vi "Z-Scan.vi"() -> ()   [LabVIEW 2020]
uses:
  <vilib>/LabVIEW Interface for Arduino/Type Defs/Board Type.ctl
  <vilib>/LabVIEW Interface for Arduino/Type Defs/Connection Type.ctl
  <vilib>/Utility/error.llb/DialogType.ctl
  <vilib>/Utility/file.llb/Write Delimited Spreadsheet (string).vi
panel:
  in  "Unidade de medida":bool
  in  "Distancia entre medidas":sgl
  out "Rodando":bool
  in  "Numero de medidas":i32
  in  "Distancia percorrida":sgl
  in  "Measurement Function (0: Period)":i32(ring)=17 items=["Period", "Frequency", "Delay", "Rise Time", "Fall Time", "Positive Duty Cycle", "Negative Duty Cycle", "Positive Pulse Width", "Negative Pulse Width", "Burst Width", "Phase", "Positive Overshoot", "Negative Overshoot", "Vpp", "Amplitude", "Voltage High", "Voltage Low", "Voltage Max", "Voltage Min", "Voltage Mean", "Voltage Mean (cycle)", "Voltage RMS", "Voltage RMS (cycle)", "Area", "Cycle Area", "Positive Edge Count", "Negative Edge Count", "Positive Pulse Count", "Negative Pulse Count", "Total Overshoot"]
  in  "Channel (0: Channel 1)":u16(ring) items=["Channel 1", "Channel 2", "Channel 3", "Channel 4", "Math", "D0", "D1", "D2", "D3", "D4", "D5", "D6", "D7", "D8", "D9", "D10", "D11", "D12", "D13", "D14", "D15", "Reference 1", "Reference 2", "Reference 3", "Reference 4", "Amplitude", "Frequency", "Phase"]
  out "Numero de paradas":sgl
  in  "Sair":bool
  out "Tabela":string[][](table)
  out "?":cluster{dbl[], dbl[]}(graph)
  out "Passos entre medidas":sgl
  out "Numero de passos":sgl
  in  "Z-Scan Automatico":bool
  in  "VISA Tektronix DPO 3052":refnum<visa-resource-name>
  in  "VISA Arduino":refnum<visa-resource-name>
  # "Não interromper a medida em andamento pelo abourt execution(canto superior esquedo), risco de dano ao motor"
  # "Para encontrar a COM: Botão Windows/ Dispositivos e impressoras/ Não especificados"
  # "Para o Software Z-Scan\n1) Selecionar a porta do dispositivo:\n  - VISA Arduino (ver a porta do USB-SERIAL CH340)\n  - Visa Tektronix (USB0::0x0699::.. do DPO 3052)\n2) Seleciona o canal do osciloscópio e o tipo de medida:\n  - Channel (ver no osciloscópio: canal 1 ou 2)\n  - Measurement Function (voltagem max)\n3) Dar RUN (canto esquerdo superior da tela)\n3) Definir os parâmetros de medida:\n  - Unidade de medida\n  - Distância percorrida (2*Z)\n  - Distância entre medidas\n  - Número de medidas (para fazer as médias)\n4) Clicla na tela para validar os dados de entrada\n5) Encontrar o foco pelas teclas direita/esquerda do teclado\n6) Clica \"Iniciar\""
  # "Para a montagem Z-Scan\n1) Conectar o osciloscópio e o arduino ao computador\n2) Ligar a fonte do arduino na tomada\n3) Girar o switch da caixinha"
  # "cm"
  # "mm"
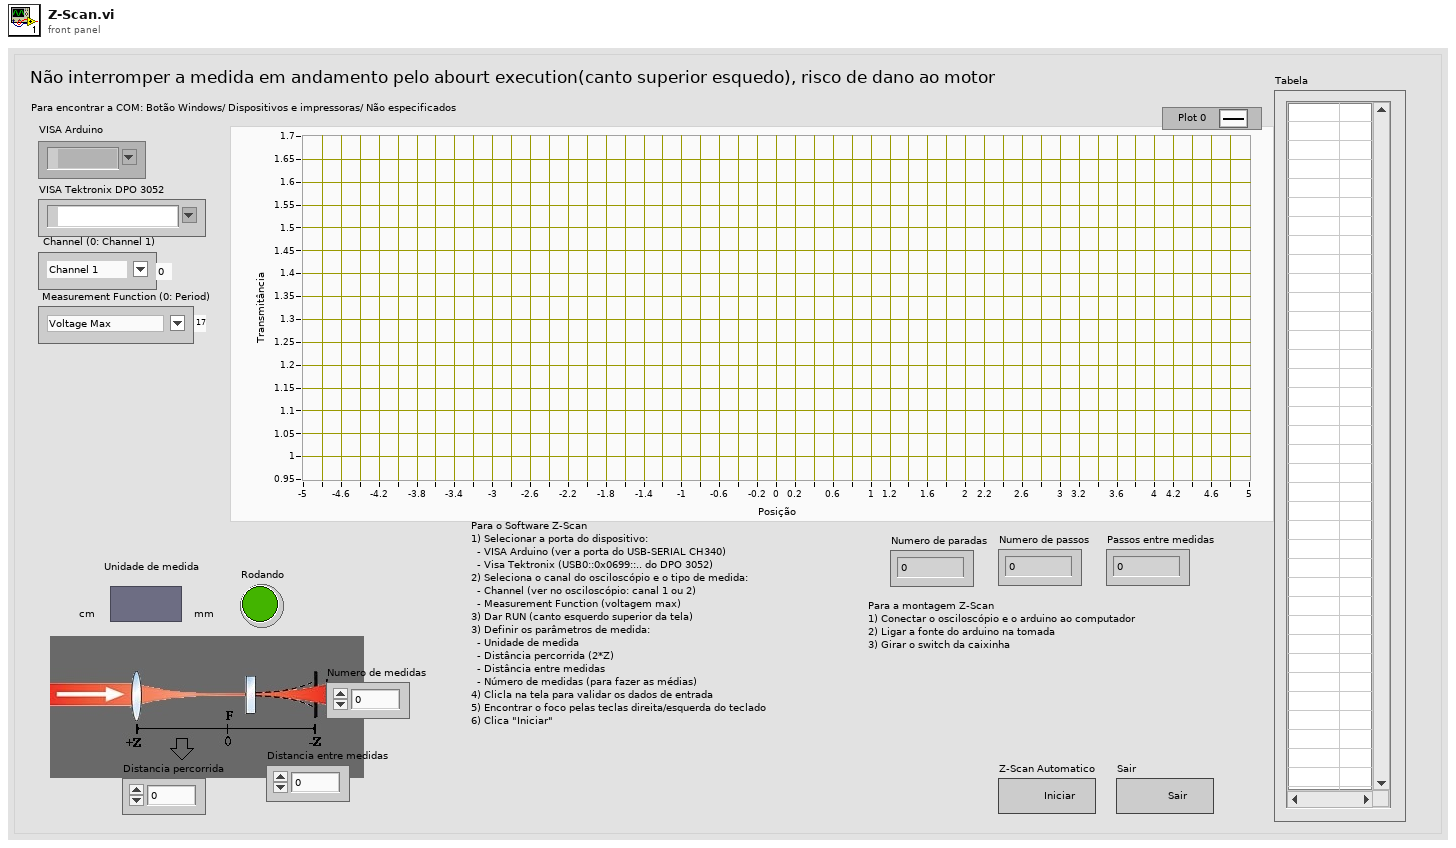
[diagram p1: front panel]
types:
  T1 = typedef "DialogType.ctl" = u16
  T2 = typedef "LabVIEW Interface for Arduino.lvlib/Connection Type.ctl" = enum8{"USB / Serial", "XBEE", "BlueSmirf (Bluetooth)"}
  T3 = typedef "LabVIEW Interface for Arduino.lvlib/Board Type.ctl" = enum16{"Uno", "Dimuelanove w/Atmega 328", "Mega 2560"}
  T4 = typedef "LabVIEW Interface for Arduino.lvlib/Arduino Resource.ctl" = cluster{"VISA resource":refnum<visa-resource-name>, "Board Type":T3, "Connection Type":enum8{"USB / Serial"}, "Bytes Per Packet (15)":u8}
  T5 = typedef "eventvkey.ctl" = enum16{"ASCII", "Enter", "Return", "Shift", "Ctrl", "Alt", "Cmd", "Opt", "Caps", "NumLock", "Clear", "Break", "Up", "Down", "Left", "Right", "Insert", "Delete", "Home", "End", "PageUp", "PageDown", "Escape", "Help", "Pause", "ScrollLock", "F1", "F2", "F3", "F4", "F5", "F6", "F7", "F8", "F9", "F10", "F11", "F12", "F13", "F14", "F15", "F16", "F17", "F18", "F19", "F20", "F21", "F22", "F23", "F24", "Play", "VolumeUp", "VolumeDown", "Mute", "Two Byte Char"}
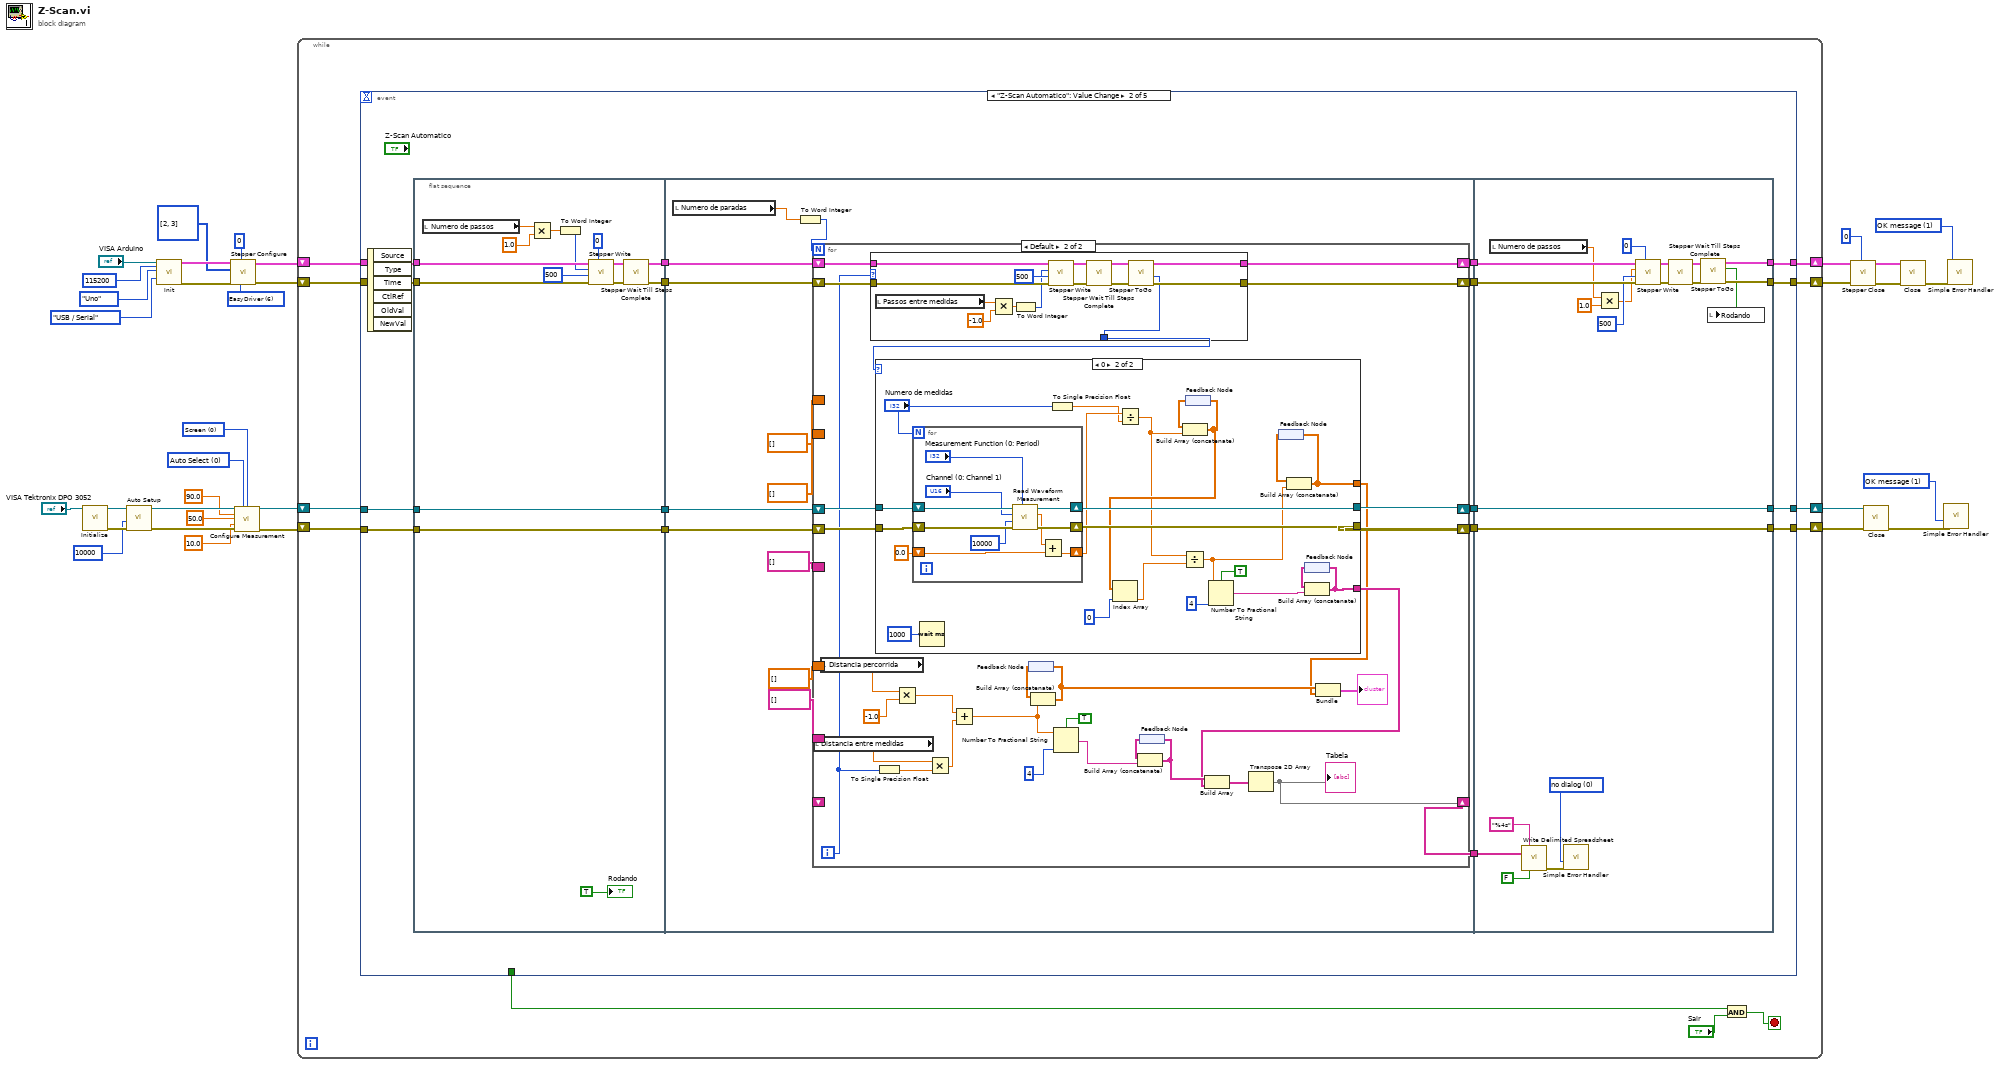
[diagram p0: block diagram]
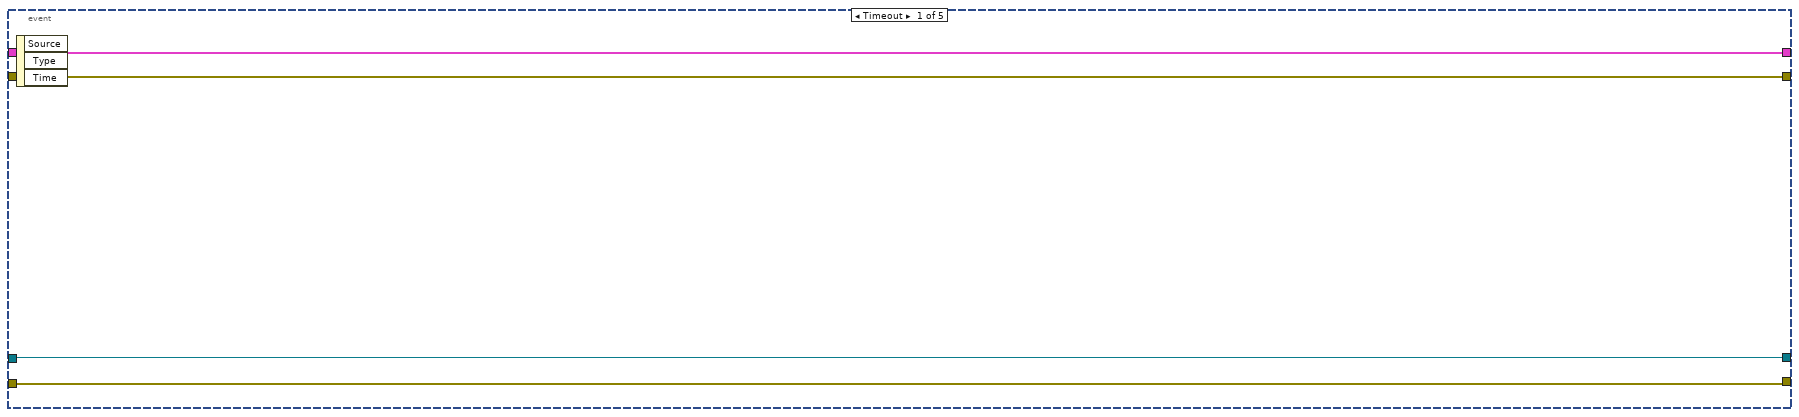
[diagram p2: hidden frame]
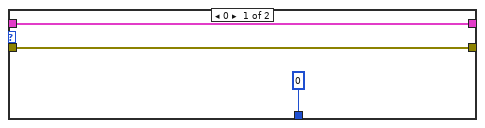
[diagram p3: hidden frame]
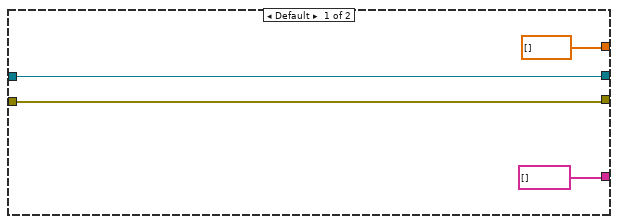
[diagram p4: hidden frame]
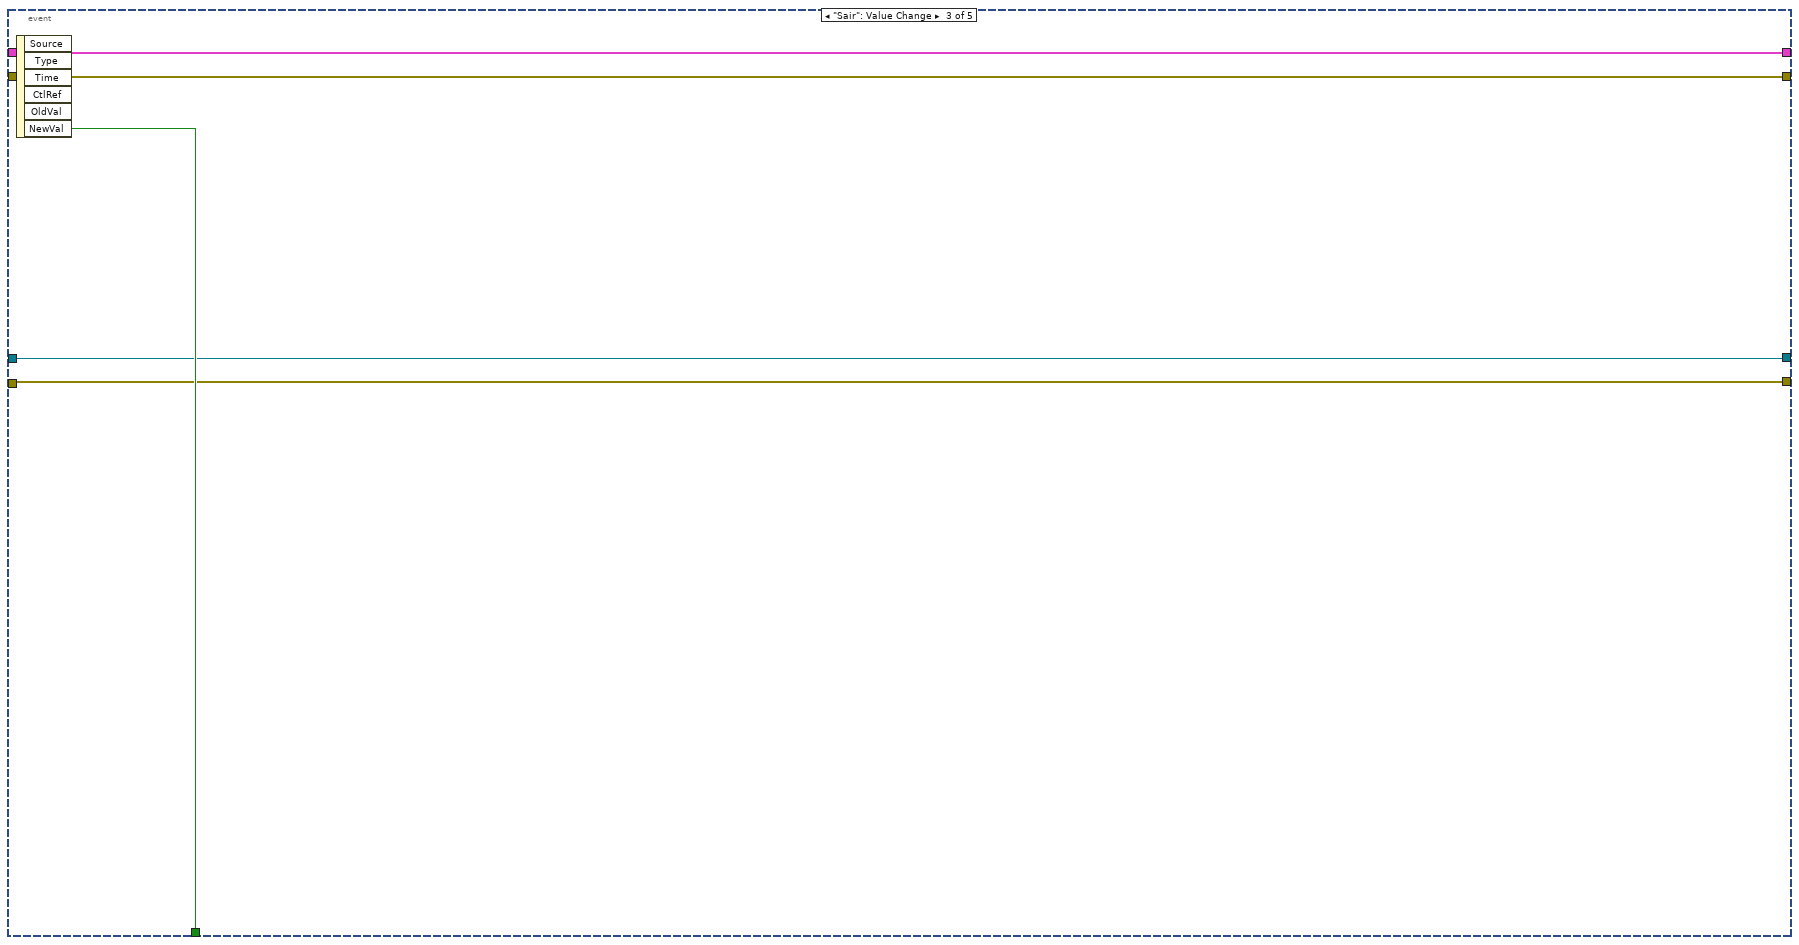
[diagram p5: hidden frame]
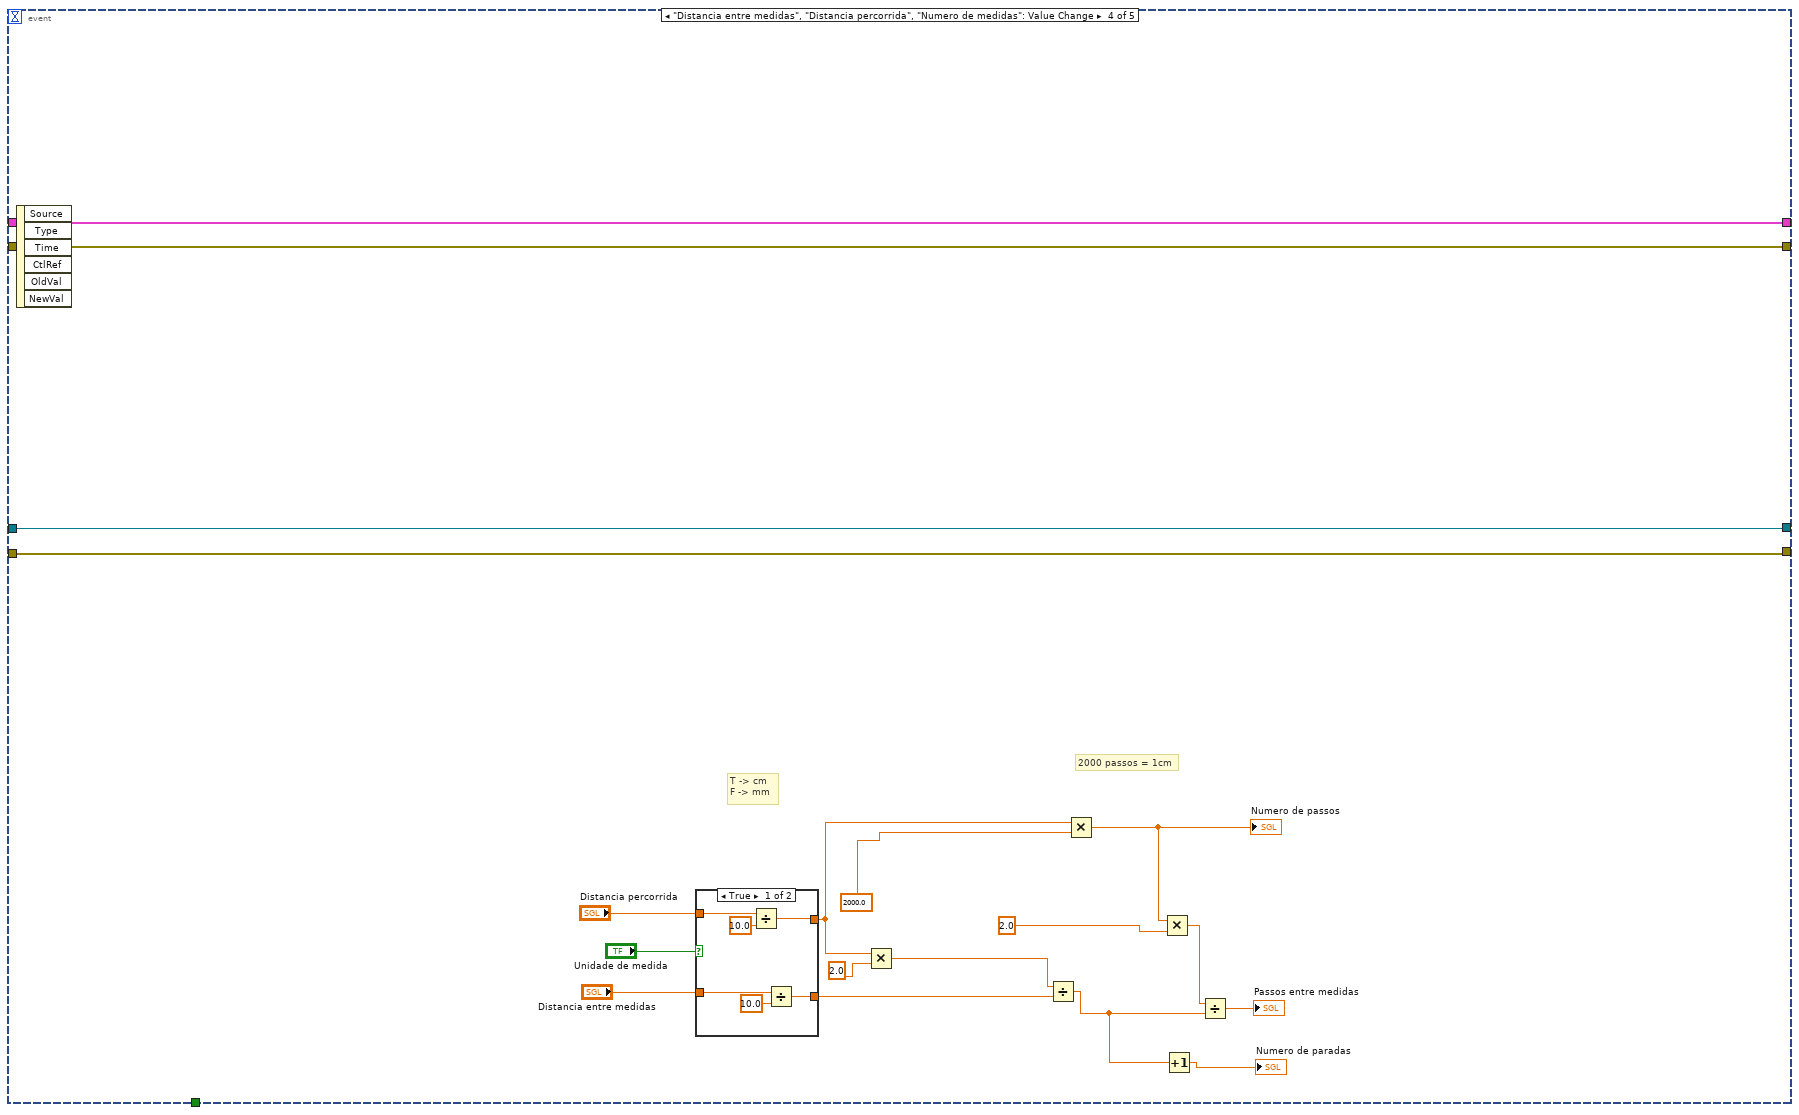
[diagram p6: hidden frame]
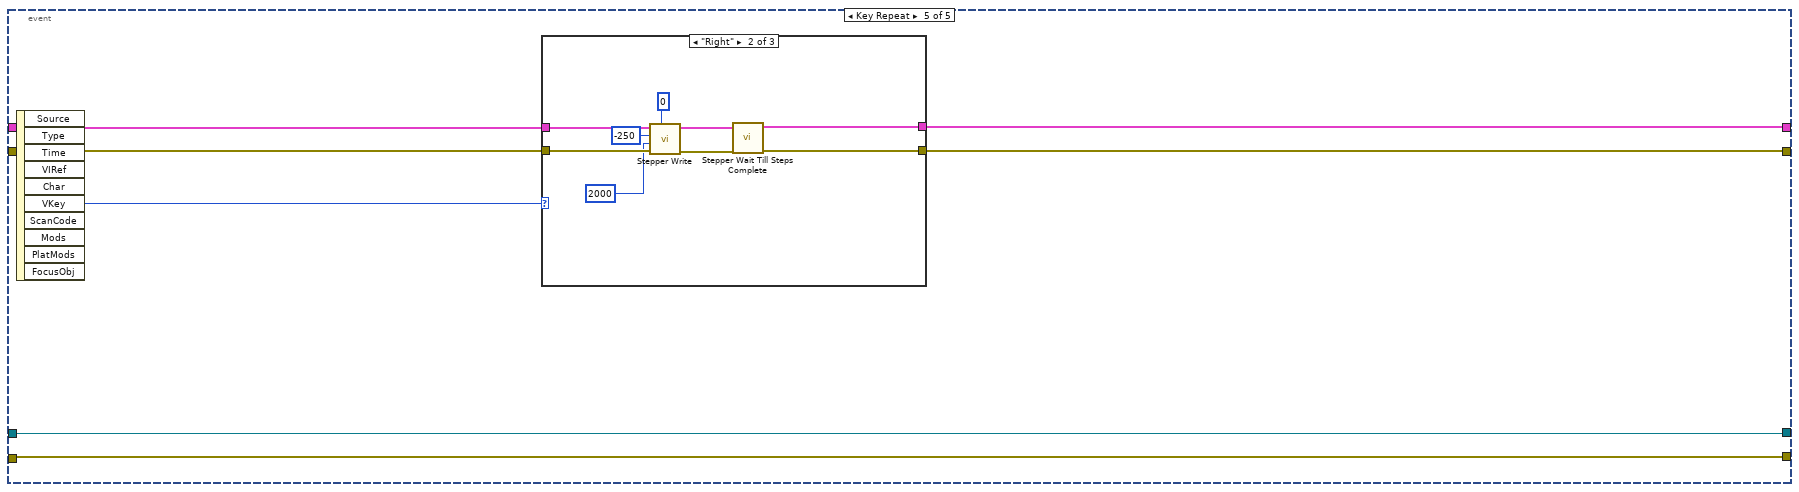
[diagram p8: hidden frame]
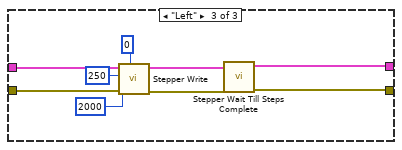
[diagram p10: hidden frame]
diagram:
  w2 = T1 1 items=["no dialog", "OK message", "continue or stop message", "OK message + warnings", "continue/stop + warnings"] ("type of dialog (OK msg:1)")
  w3 = T1 1 items=["no dialog", "OK message", "continue or stop message", "OK message + warnings", "continue/stop + warnings"] ("type of dialog (OK msg:1)")
  w17 = u16 0 items=["Screen", "Between Cursors", "Off"] ("Gating (0: Screen)")
  w18 = 0 items=["Auto Select", "Histogram", "Min/Max"] ("Ref Level Calculate Method (0: Auto Select)")
  w28 = u8 6 items=["2 Wire (Pulse & Direction)"=1, "2 Wire"=2, "4 Wire"=4, "EasyDriver"=6, "AF Motor Shield (Stepper 1 & 2 Only)"=5] ("Control Method")
  n1 = call <instrlib>:"Initialize.vi"("VISA resource name"="VISA Tektronix DPO 3052") -> ("error out"=w23:errorcluster, "VISA resource name out"=w22:refnum<visa-resource-name>)  [unwired: 9 in]
  n2 = call <instrlib>:"Auto Setup.vi"("error in (no error)"=w23, "Maximum Time (10000ms)"=10000, "VISA resource name"=w22) -> ("error out"=w19:errorcluster, "VISA resource name out"=w20:refnum<visa-resource-name>)  [unwired: 7 in]
  n3 = call <vilib>:"Init.vi"("VISA resource"="VISA Arduino", "Baud Rate (115200)"=u32 115200, "Board Type (Uno)"=Board_Type."Uno", "Connection Type (USB/Serial)"=Connection_Type."USB / Serial") -> ("Arduino Resource"=w34:T4, "error out"=w35:errorcluster)  [unwired: 14 in]
  n4 = call <vilib>:"Stepper Configure.vi"("Control Method"=w28, "Stepper #"=u8 0, "error in"=w35, "Stepper Pins"=u8[] [2, 3], "Arduino Resource"=w34) -> ("error out"=w25:errorcluster, "Arduino Resource Out"=w26:T4)  [unwired: 5 in]
  n5 = call <instrlib>:"Configure Measurement.vi"("VISA resource name"=w20, "Ref Level Calculate Method (0: Auto Select)"=w18, "Gating (0: Screen)"=w17, "High Ref (90%)"=90.0, "Mid Ref (50%)"=50.0, "Low Ref (10%)"=10.0, "error in (no error)"=w19) -> ("VISA resource name out"=w13:refnum<visa-resource-name>, "error out"=w12:errorcluster)  [unwired: 7 in]
  n6 = while {
    shift-right: [w42] -> w9
    shift-left: w26 -> [w46]
    shift-right: [w41] -> w8
    shift-left: w25 -> [w45]
    shift-right: [w40] -> w7
    shift-left: w13 -> [w44]
    shift-right: [w39] -> w6
    shift-left: w12 -> [w43]
    stop <- w36 stop-if-true
    n7 = event shown="[1] \"Z-Scan Automatico\": Value Change" {
      selector: _ -> [_ _ _ _ _]
      dyn-events: _ -> [_ _ _ _ _]
      timeout: _ -> [_ _ _ _ _]
      tunnel: w46 -> [w47 w67 w202 w211 w236]
      tunnel: w45 -> [w48 w66 w203 w212 w235]
      tunnel: w44 -> [w49 w58 w204 w213 w239]
      tunnel: w43 -> [w50 w56 w205 w214 w238]
      tunnel: [w47 w61 w202 w211 w234] -> w42
      tunnel: [w48 w60 w203 w212 w233] -> w41
      tunnel: [w49 w55 w204 w213 w239] -> w40
      tunnel: [w50 w52 w205 w214 w238] -> w39
      tunnel: [_ _ w206 _ _] -> w37
      event Timeout {
        n8 = event-data() -> ()  [unwired: 1 in, 3 out]
      }
      event "Z-Scan Automatico": Value Change {
        n9 = event-data() -> ()  [unwired: 1 in, 6 out]
        n10 = flat-sequence {
          tunnel: w67 -> [w80]
          tunnel: w66 -> [w79]
          tunnel: [w78] -> w65
          tunnel: [w77] -> w64
          tunnel: [w76] -> w59
          tunnel: w58 -> [w76]
          tunnel: [w75] -> w57
          tunnel: w56 -> [w75]
          tunnel: w65 -> [w98]
          tunnel: w64 -> [w97]
          tunnel: [w96] -> w63
          tunnel: [w95] -> w62
          tunnel: w59 -> [w94]
          tunnel: w57 -> [w93]
          tunnel: [w92] -> w54
          tunnel: [w91] -> w53
          tunnel: [w86] -> w51
          tunnel: w63 -> [w199]
          tunnel: w62 -> [w198]
          tunnel: [w182] -> w61
          tunnel: [w183] -> w60
          tunnel: [w197] -> w55
          tunnel: w54 -> [w197]
          tunnel: [w196] -> w52
          tunnel: w53 -> [w196]
          tunnel: w51 -> [w190]
          frame #0 {
            n11 = local read "Numero de passos"() -> (w70:sgl)
            n12 = Multiply(x=w70, y=1.0) -> (x*y=w69:dbl)
            n13 = To Word Integer(number=w69) -> (16bit integer=w68:i16)
            n14 = call <vilib>:"Stepper Write.vi"("Stepper #"=u8 0, "error in"=w79, "Set Speed (Steps per Second)"=i16 500, "# of Steps to Move"=w68, "Arduino Resource"=w80) -> ("error out"=w81:errorcluster, "Arduino Resource Out"=w82:T4)  [unwired: 5 in]
            n15 = call <vilib>:"Stepper Wait Till Steps Complete.vi"("error in"=w81, "Arduino Resource In"=w82) -> ("error out"=w77:errorcluster, "Arduino Resource Out"=w78:T4)  [unwired: 8 in]
            "Rodando" <- TRUE ("Rodando?")
          }
          frame #1 {
            n16 = local read "Numero de paradas"() -> (w83:sgl)
            n17 = To Word Integer(number=w83) -> (16bit integer=w84:i16)
            n18 = for {
              N: w84 -> [_]
              shift-right: [w124] -> w95
              shift-left: w97 -> [w126]
              shift-right: [w125] -> w96
              shift-left: w98 -> [w127]
              shift-right: [w120] -> w92
              shift-left: w94 -> [w122]
              shift-right: [w119] -> w91
              shift-left: w93 -> [w121]
              border: dbl[] [] -> [_]
              border: dbl[] [] -> [_]
              border: dbl[] [] -> [_]
              border: string[] [] -> [_]
              shift-right: [w101] -> w86
              shift-left: _ -> [_]
              border: string[] [] -> [_]
              i -> [w99]
              n19 = local read "Distancia entre medidas"() -> (w106:sgl)
              n20 = local read "Distancia percorrida"() -> (w117:sgl)
              n21 = case shown="Default" w99 {
                tunnel: w127 -> [w129 w142]
                tunnel: w126 -> [w130 w141]
                tunnel: [w129 w138] -> w125
                tunnel: [w130 w137] -> w124
                tunnel: [u16 0 ("Steps remaining") w136] -> w123
                frame 0 {
                }
                frame Default {
                  n22 = local read "Passos entre medidas"() -> (w134:sgl)
                  n23 = Multiply(x=w134, y=sgl -1.0) -> (x*y=w132:sgl)
                  n24 = To Word Integer(number=w132) -> (16bit integer=w131:i16)
                  n25 = call <vilib>:"Stepper Write.vi"("error in"=w141, "Set Speed (Steps per Second)"=i16 500, "# of Steps to Move"=w131, "Arduino Resource"=w142) -> ("error out"=w144:errorcluster, "Arduino Resource Out"=w143:T4)  [unwired: 6 in]
                  n26 = call <vilib>:"Stepper Wait Till Steps Complete.vi"("error in"=w144, "Arduino Resource In"=w143) -> ("error out"=w140:errorcluster, "Arduino Resource Out"=w139:T4)  [unwired: 8 in]
                  n27 = call <vilib>:"Stepper ToGo.vi"("error in"=w140, "Arduino Resource"=w139) -> ("error out"=w137:errorcluster, "Steps remaining"=w136:u16, "Arduino Resource Out"=w138:T4)  [unwired: 6 in, 1 out]
                }
              }
              n28 = case shown="0" w123 {
                tunnel: w122 -> [w148 w168]
                tunnel: w121 -> [w147 w166]
                tunnel: [w148 w167] -> w120
                tunnel: [w147 w165] -> w119
                tunnel: [dbl[] [] w169] -> w102
                tunnel: [string[] [] w159] -> w103
                frame Default {
                }
                frame 0 {
                  n29 = for {
                    N: "Numero de medidas" -> [_]
                    shift-right: [w179] -> w167
                    shift-left: w168 -> [w180]
                    shift-right: [w177] -> w165
                    shift-left: w166 -> [w178]
                    shift-right: [w174] -> w163
                    shift-left: 0.0 -> [w173]
                    n30 = call <instrlib>:"Read Waveform Measurement.vi"("Measurement Function (0: Period)"="Measurement Function (0: Period)", "error in (no error)"=w178, "Maximum Time (10000ms)"=u32 10000, "Channel (0: Channel 1)"="Channel (0: Channel 1)", "VISA resource name"=w180) -> ("error out"=w177:errorcluster, "Measurement Value"=w175:dbl, "VISA resource name out"=w179:refnum<visa-resource-name>)  [unwired: 4 in]
                    n31 = Add(x=w175, y=w173) -> (x+y=w174:dbl)
                  }
                  n32 = Wait (ms)(milliseconds to wait=u32 1000) -> ()  [unwired: 1 out]
                  n33 = To Single Precision Float(number="Numero de medidas") -> (single precision float=w150:sgl)
                  n34 = Divide(x=w163, y=w150) -> (x/y=w152:dbl)
                  n35 = feedback #1() -> (w156:dbl[])
                  n36 = Build Array (concatenate)(w156, w152) -> (w153:dbl[])
                  n37 = Index Array(array=w153, index=0) -> (element=w155:dbl)
                  n38 = Divide(x=w152, y=w155) -> (x/y=w157:dbl)
                  n39 = feedback-in #1(w153) -> ()
                  n40 = Number To Fractional String(use system decimal point (T)=TRUE, number=w157, precision (6)=i16 4 ("width (-)")) -> (F-format string=w158:string)  [unwired: 1 in]
                  n41 = feedback #2() -> (w170:dbl[])
                  n42 = Build Array (concatenate)(w170, w157) -> (w169:dbl[])
                  n43 = feedback-in #2(w169) -> ()
                  n44 = feedback #3() -> (w160:string[])
                  n45 = Build Array (concatenate)(w160, w158) -> (w159:string[])
                  n46 = feedback-in #3(w159) -> ()
                }
              }
              n47 = To Single Precision Float(number=w99) -> (single precision float=w100:sgl)
              n48 = Multiply(x=w117, y=-1.0) -> (x*y=w116:dbl)
              n49 = Multiply(x=w106, y=w100) -> (x*y=w115:sgl)
              n50 = Add(x=w116, y=w115) -> (x+y=w111:dbl)
              n51 = feedback #4() -> (w108:dbl[])
              n52 = Build Array (concatenate)(w108, w111) -> (w107:dbl[])
              n53 = feedback-in #4(w107) -> ()
              n54 = Number To Fractional String(use system decimal point (T)=TRUE, number=w111, precision (6)=i16 4 ("width (-)")) -> (F-format string=w109:string)  [unwired: 1 in]
              n55 = feedback #5() -> (w114:string[])
              n56 = Build Array (concatenate)(w114, w109) -> (w113:string[])
              n57 = feedback-in #5(w113) -> ()
              n58 = Build Array(w113, w103) -> (w105:string[][])
              n59 = Transpose 2D Array(2D array=w105) -> (transposed array=w101:string[][])
              "Tabela" <- w101
              n60 = Bundle(w107, w102) -> (→"?":cluster{dbl[], dbl[]})  [unwired: 1 in]
            }
          }
          frame #2 {
            w186 = T1 0 items=["no dialog", "OK message", "continue or stop message", "OK message + warnings", "continue/stop + warnings"] ("type of dialog (OK msg:1)")
            n61 = local read "Numero de passos"() -> (w192:sgl)
            n62 = call-poly <vilib>:"Write Delimited Spreadsheet.vi"("format (%s)"="%4s", "2D data"=w190, "transpose? (no:F)"=FALSE) -> ("error out"=w187:errorcluster)  [unwired: 11 in, 1 out]
            n63 = call <vilib>:"Simple Error Handler.vi"("type of dialog (OK msg:1)"=w186, "error in (no error)"=w187) -> ()  [unwired: 3 in, 5 out]
            n64 = Multiply(x=w192, y=1.0) -> (x*y=w191:dbl)
            n65 = call <vilib>:"Stepper Write.vi"("Stepper #"=u8 0, "error in"=w198, "Set Speed (Steps per Second)"=i16 500, "# of Steps to Move"=w191, "Arduino Resource"=w199) -> ("error out"=w200:errorcluster, "Arduino Resource Out"=w201:T4)  [unwired: 5 in]
            n66 = call <vilib>:"Stepper Wait Till Steps Complete.vi"("error in"=w200, "Arduino Resource In"=w201) -> ("error out"=w185:errorcluster, "Arduino Resource Out"=w184:T4)  [unwired: 8 in]
            n67 = call <vilib>:"Stepper ToGo.vi"("error in"=w185, "Arduino Resource"=w184) -> ("error out"=w183:errorcluster, "Steps Remaining?"=w181:bool, "Arduino Resource Out"=w182:T4)  [unwired: 6 in, 1 out]
            n68 = local write "Rodando"(w181) -> ()
          }
        }
      }
      event "Sair": Value Change {
        n69 = event-data() -> ("NewVal"=w206:bool)  [unwired: 1 in, 5 out]
      }
      event "Distancia entre medidas", "Distancia percorrida", "Numero de medidas": Value Change {
        # "T -> cm\nF -> mm"
        # "2000 passos = 1cm"
        n70 = event-data() -> ()  [unwired: 1 in, 6 out]
        n71 = case shown="True" "Unidade de medida" {
          tunnel: [w228 w232] -> w209
          tunnel: [w227 w231] -> w221
          tunnel: "Distancia percorrida" -> [w230 w232]
          tunnel: "Distancia entre medidas" -> [w229 w231]
          frame True {
            n72 = Divide(x=w230, y=sgl 10.0) -> (x/y=w228:sgl)
            n73 = Divide(x=w229, y=sgl 10.0) -> (x/y=w227:sgl)
          }
          frame False {
          }
        }
        n74 = Multiply(x=w209, y=2.0) -> (x*y=w219:dbl)
        n75 = Divide(x=w219, y=w221) -> (x/y=w208:dbl)
        n76 = Multiply(x=w209, y=sgl 2000.0) -> (x*y=w217:sgl)
        "Numero de passos" <- w217
        n77 = Multiply(x=w217, y=sgl 2.0) -> (x*y=w218:sgl)
        n78 = Increment(x=w208) -> (x+1=→"Numero de paradas":dbl)
        n79 = Divide(x=w218, y=w208) -> (x/y=→"Passos entre medidas":dbl)
      }
      event Key Repeat {
        n80 = event-data() -> ("VKey"=w237:T5)  [unwired: 1 in, 9 out]
        n81 = case shown="\"Right\"" w237 {
          tunnel: w236 -> [w241 w250 w259]
          tunnel: w235 -> [w240 w249 w256]
          tunnel: [w241 w246 w257] -> w234
          tunnel: [w240 w245 w254] -> w233
          frame "ASCII", Default {
          }
          frame "Right" {
            n82 = call <vilib>:"Stepper Write.vi"("Stepper #"=u8 0, "error in"=w249, "Set Speed (Steps per Second)"=i16 2000, "# of Steps to Move"=i16 -250, "Arduino Resource"=w250) -> ("error out"=w247:errorcluster, "Arduino Resource Out"=w248:T4)  [unwired: 5 in]
            n83 = call <vilib>:"Stepper Wait Till Steps Complete.vi"("error in"=w247, "Arduino Resource In"=w248) -> ("error out"=w245:errorcluster, "Arduino Resource Out"=w246:T4)  [unwired: 8 in]
          }
          frame "Left" {
            n84 = call <vilib>:"Stepper Write.vi"("Stepper #"=u8 0, "error in"=w256, "Set Speed (Steps per Second)"=i16 2000, "# of Steps to Move"=i16 250, "Arduino Resource"=w259) -> ("error out"=w255:errorcluster, "Arduino Resource Out"=w258:T4)  [unwired: 5 in]
            n85 = call <vilib>:"Stepper Wait Till Steps Complete.vi"("error in"=w255, "Arduino Resource In"=w258) -> ("error out"=w254:errorcluster, "Arduino Resource Out"=w257:T4)  [unwired: 8 in]
          }
        }
      }
    }
    n86 = And(x=w37, y="Sair") -> (x .and. y?=w36:bool)
  }
  n87 = call <vilib>:"Stepper Close.vi"("Stepper #"=u8 0, "error in"=w8, "Arduino Resource"=w9) -> ("error out"=w11:errorcluster, "Arduino Resource Out"=w10:T4)  [unwired: 7 in]
  n88 = call <instrlib>:"Close.vi"("error in (no error)"=w6, "VISA resource name"=w7) -> ("error out"=w4:errorcluster)  [unwired: 9 in]
  n89 = call <instrlib>:"Close.vi"("Arduino Resource"=w10, "error in"=w11) -> ("error out"=w5:errorcluster)  [unwired: 13 in]
  n90 = call <vilib>:"Simple Error Handler.vi"("type of dialog (OK msg:1)"=w3, "error in (no error)"=w4) -> ()  [unwired: 3 in, 5 out]
  n91 = call <vilib>:"Simple Error Handler.vi"("type of dialog (OK msg:1)"=w2, "error in (no error)"=w5) -> ()  [unwired: 3 in, 5 out]
